vi "S2C_ExeScriptFailResultRoute.vi"(8 "Error In":errorcluster, 10 "LastStep?":bool, 11 "Q_Ref":refnum<queue>) -> (0 "Error Out":errorcluster, 3 "IncRow?":bool)   [LabVIEW 2015]
doc: "Update the results cell in the execution table for the currently executing line item, and determines the next step to take in the execution."
uses:
  Globals/S2C_Globals.vi
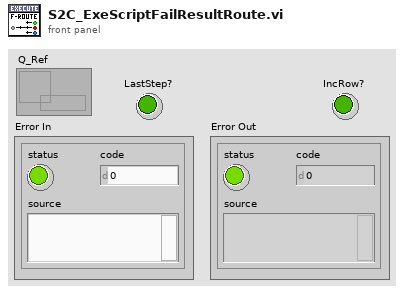
[diagram p1: front panel]
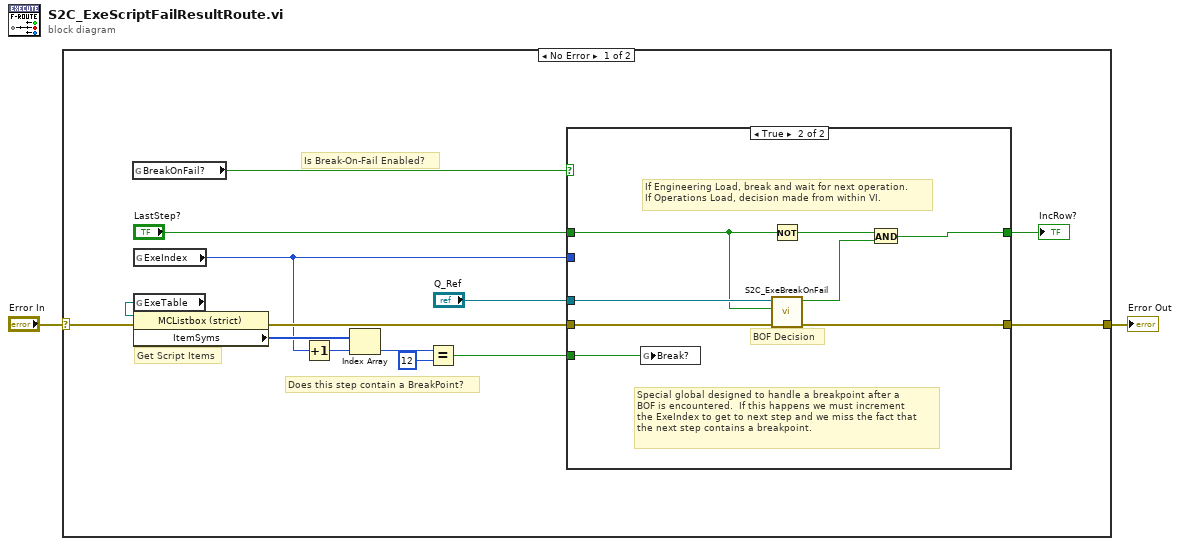
[diagram p0: block diagram]
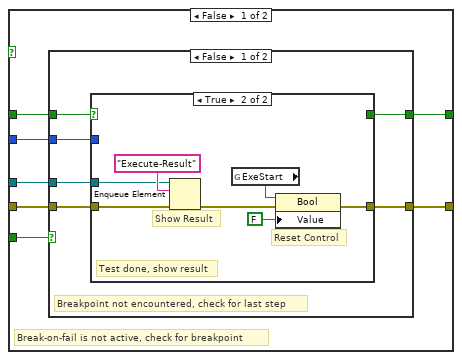
[diagram p2: hidden frame]
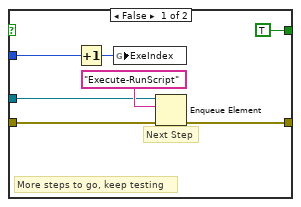
[diagram p3: hidden frame]
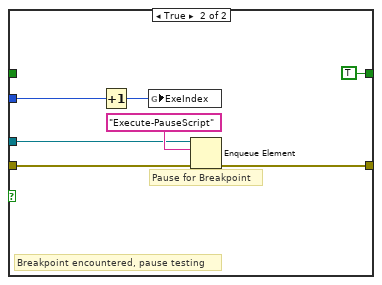
[diagram p4: hidden frame]
diagram:
  n1 = case shown="No Error" "Error In" {
    selector: "Error In" -> [w9 w59]
    tunnel: [w15 w59] -> w1
    frame No Error {
      # "Is Break-On-Fail Enabled?"
      # "Does this step contain a BreakPoint?"
      # "Get Script Items"
      n2 = global read "S2C_Globals.vi" "BreakOnFail?"() -> (w7:bool)
      n3 = global read "S2C_Globals.vi" "ExeIndex"() -> (w4:i32)
      n4 = global read "S2C_Globals.vi" "ExeTable"() -> (w10:refnum<vi>)
      n5 = property class="MCListbox (strict)"(reference=w10, error in=w9) -> (error out=w8:errorcluster, "ItemSyms"=w5:i32[])  [unwired: 1 out]
      n6 = Increment(x=w4) -> (x+1=w13:i32)
      n7 = Index Array(array=w5, index=w13) -> (element=w11:i32)
      n8 = Equal?(x=w11, y=12) -> (x = y?=w3:bool)
      n9 = case shown="True" w7 {
        tunnel: "Q_Ref" -> [w23 w56]
        tunnel: [w22 w57] -> w15
        tunnel: "LastStep?" -> [w21 w51]
        tunnel: w4 -> [w20 _]
        tunnel: w8 -> [w19 w58]
        tunnel: w3 -> [w18 w55]
        tunnel: [w17 w53] -> w6
        frame False {
          # "Break-on-fail is not active, check for breakpoint"
          n10 = case shown="False" w18 {
            tunnel: w20 -> [w27 w46]
            tunnel: w19 -> [w29 w49]
            tunnel: [w28 w48] -> w22
            tunnel: w23 -> [w26 w47]
            tunnel: w21 -> [w25 _]
            tunnel: [w24 TRUE] -> w17
            frame False {
              # "Breakpoint not encountered, check for last step"
              n11 = case shown="True" w25 {
                tunnel: w29 -> [w36 w39]
                tunnel: [w35 w37] -> w28
                tunnel: w27 -> [w32 _]
                tunnel: w26 -> [w31 w38]
                tunnel: [TRUE _] -> w24
                frame False {
                  # "More steps to go, keep testing"
                  # "Next Step"
                  n12 = Increment(x=w32) -> (x+1=w33:i32)
                  n13 = global write "S2C_Globals.vi" "ExeIndex"(w33) -> ()
                  n14 = Enqueue Element(queue=w31, element="Execute-RunScript", error in (no error)=w36) -> (error out=w35:errorcluster)  [unwired: 1 in, 2 out]
                }
                frame True {
                  # "Test done, show result"
                  # "Show Result"
                  # "Reset Control"
                  n15 = Enqueue Element(queue=w38, element="Execute-Result", error in (no error)=w39) -> (error out=w41:errorcluster)  [unwired: 1 in, 2 out]
                  n16 = global read "S2C_Globals.vi" "ExeStart"() -> (w43:refnum<vi>)
                  n17 = property class="Bool"(reference=w43, error in=w41, "Value"=FALSE) -> (error out=w37:errorcluster)  [unwired: 1 out]
                }
              }
            }
            frame True {
              # "Breakpoint encountered, pause testing"
              # "Pause for Breakpoint"
              n18 = Increment(x=w46) -> (x+1=w45:i32)
              n19 = global write "S2C_Globals.vi" "ExeIndex"(w45) -> ()
              n20 = Enqueue Element(queue=w47, element="Execute-PauseScript", error in (no error)=w49) -> (error out=w48:errorcluster)  [unwired: 1 in, 2 out]
            }
          }
        }
        frame True {
          # "Special global designed to handle a breakpoint after a\nBOF is encountered.  If this happens we must increment\nthe ExeIndex to get to next step and we miss the fact that\nthe next step contains a breakpoint."
          # "If Engineering Load, break and wait for next operation.\nIf Operations Load, decision made from within VI."
          # "BOF Decision"
          n21 = global write "S2C_Globals.vi" "Break?"(w55) -> ()
          n22 = Not(x=w51) -> (.not. x?=w52:bool)
          n23 = call "S2C_ExeBreakOnFail.vi"("Error In"=w58, "LastStep?"=w51, "Q_Ref"=w56) -> ("Error Out"=w57:errorcluster, "IncRow?"=w54:bool)  [unwired: 7 in]
          n24 = And(x=w52, y=w54) -> (x .and. y?=w53:bool)
        }
      }
      "IncRow?" <- w6
    }
    frame Error {
    }
  }
  "Error Out" <- w1
